vi "Vision Research Phantom Series Utility Clean Up Initialize.vi"(11 "Error In (no error)":errorcluster) -> (15 "Error Out":errorcluster)   [LabVIEW 2013, in "VRI.lvlib"]
doc: "This Utility VI closes any open VISA sessions in the event that there is an error during an initialization. It is called only from the Vision Research Phantom Series Initialize VI, and is not meant to be altered. Changing this VI can cause the Vision Research Phantom Series Initialize VI to operate improperly.\n\nWritten by:\nBLOOMY CONTROLS, INC\nWINDSOR, CT 06095, USA\n860-298-9925\nwww.bloomy.com\nV1.0.0\nMay, 2004"
uses:
  VRI.lvlib
panel:
  # "For instructions on the use of this VI, press Ctrl+H to display the help window and move the mouse over the icon, controls, and indicators"
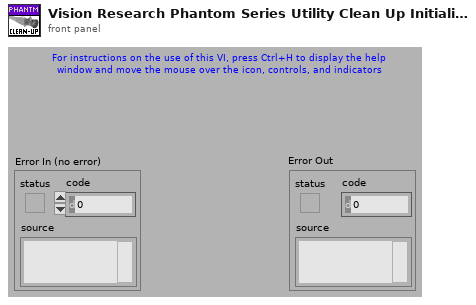
[diagram p1: front panel]
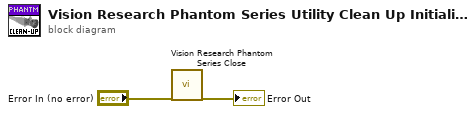
[diagram p0: block diagram]
diagram:
  n1 = call "Vision Research Phantom Series Close.vi"("Error In (no error)"="Error In (no error)") -> ("Error Out"=→"Error Out":errorcluster)  [unwired: 18 out]
